vi "get preset2 name.vi"() -> (0 "Preset name out":string)   [LabVIEW 2019]
panel:
  in  "OK Button":bool
  in  "Preset name":string
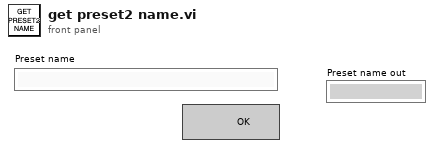
[diagram p1: front panel]
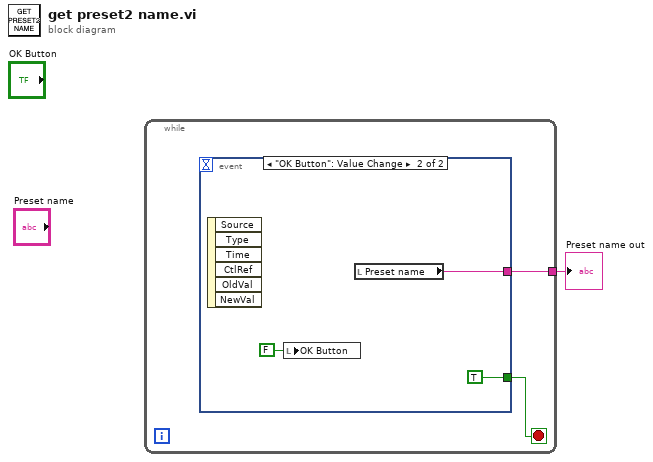
[diagram p0: block diagram]
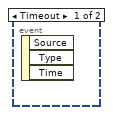
[diagram p2: hidden frame]
diagram:
  n1 = while {
    tunnel: [w3] -> w1
    stop <- w2 stop-if-true
    n2 = event shown="[1] \"OK Button\": Value Change" {
      selector: _ -> [_ _]
      dyn-events: _ -> [_ _]
      timeout: _ -> [_ _]
      tunnel: [_ w5] -> w3
      tunnel: [_ TRUE] -> w2
      event Timeout {
        n3 = event-data() -> ()  [unwired: 1 in, 3 out]
      }
      event "OK Button": Value Change {
        n4 = event-data() -> ()  [unwired: 1 in, 6 out]
        n5 = local write "OK Button"(FALSE ("OK Button")) -> ()
        n6 = local read "Preset name"() -> (w5:string)
      }
    }
  }
  "Preset name out" <- w1
